vi "GetCursors.vi"(11 "WaveformGraph in":refnum<vi>) -> (3 "Cursor Positions":dbl[](array[numeric]))   [LabVIEW 2020]
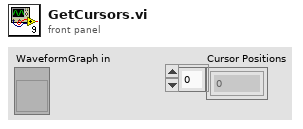
[diagram p1: front panel]
types:
  T1 = typedef "LVCursorListTypeDef.ctl" = cluster{"Name":string, "Color":u32, "Style":u8, "Point Style":u8, "Name Visible":bool, "Allow Drag":bool, "Cursor Mode":u32, "Plot":i32, "Index":i32, "Position":cluster{"X":dbl, "Y":dbl}, "X Scale":u32, "Y Scale":u32, "Watch Plots":i32[], "Watch All Plots":bool, "Plot Area":i32, "Label Offset":cluster{"X":dbl, "Y":dbl}}[]
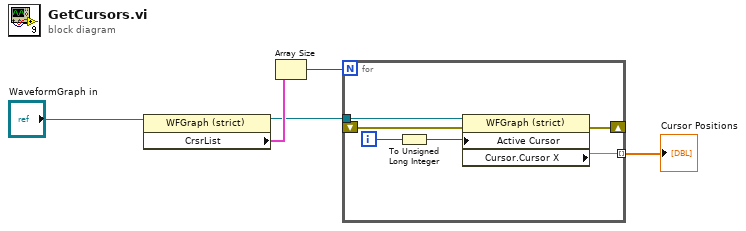
[diagram p0: block diagram]
diagram:
  n1 = property class="WFGraph (strict)"(reference="WaveformGraph in") -> (reference out=w1:refnum<vi>, "CrsrList"=w2:T1)  [unwired: 1 in, 1 out]
  n2 = Array Size(array=w2) -> (size(s)=w3:i32)
  n3 = for {
    N: w3 -> [_]
    tunnel: w1 -> [w11]
    tunnel: [w10] -> w5 mode=indexing
    shift-right: [w9] -> _
    shift-left: _ -> [w8]
    i -> [w7]
    n4 = To Unsigned Long Integer(number=w7) -> (unsigned 32bit integer=w6:u32)
    n5 = property class="WFGraph (strict)"(reference=w11, error in=w8, "Active Cursor"=w6) -> (error out=w9:errorcluster, "Cursor.Cursor X"=w10:dbl)  [unwired: 1 out]
  }
  "Cursor Positions" <- w5
